vi "CreateNamesArrayCMP.vi"(11 "Cluster":T1) -> (3 "Array":string[](array[string]))   [LabVIEW 2014]
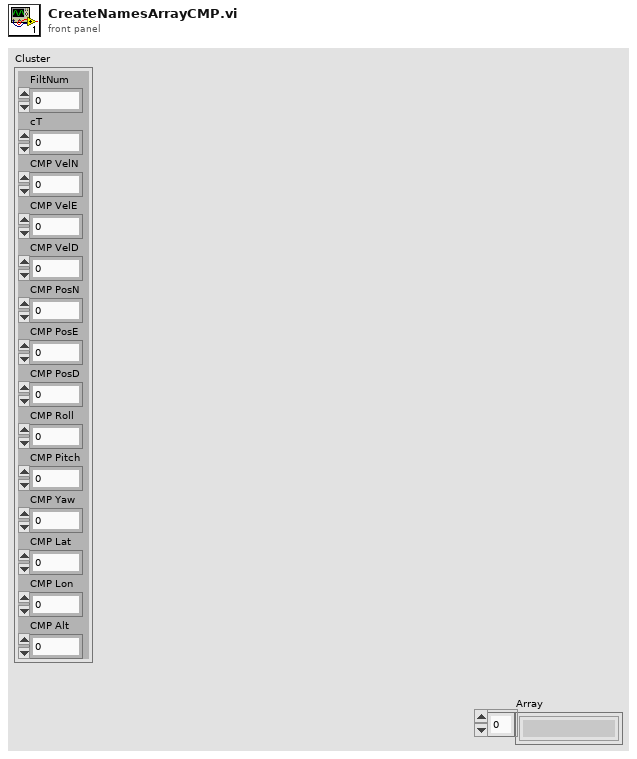
[diagram p1: front panel]
types:
  T1 = cluster{"FiltNum":i32, "cT":dbl, "CMP VelN":sgl, "CMP VelE":sgl, "CMP VelD":sgl, "CMP PosN":sgl, "CMP PosE":sgl, "CMP PosD":sgl, "CMP Roll":sgl, "CMP Pitch":sgl, "CMP Yaw":sgl, "CMP Lat":dbl, "CMP Lon":dbl, "CMP Alt":sgl}
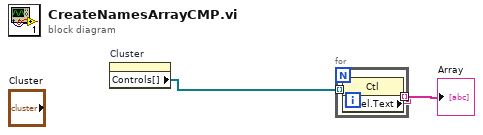
[diagram p0: block diagram]
diagram:
  n1 = property on="Cluster" class="Clust (strict)"() -> ("Controls[]"=w1:refnum<vi>[])  [unwired: 2 in, 2 out]
  n2 = for {
    tunnel: w1 -> [w4] mode=indexing
    tunnel: [w3] -> w2 mode=indexing
    n3 = property class="Ctl"(reference=w4) -> ("Label.Text"=w3:string)  [unwired: 1 in, 2 out]
  }
  "Array" <- w2
